vi "Read tag.vi"(8 "error in (no error)":errorcluster, 11 "current tag file io module runtime in":refnum<class "current tag file io module runtime.lvclass">) -> (0 "error out":errorcluster, 2 "tag":T1[](array[typedef]), 3 "current tag file io module runtime out":refnum<class "current tag file io module runtime.lvclass">)   [LabVIEW 2013, in "current tag file io module runtime.lvclass"]
uses:
  current tag file io module runtime.lvclass
  current tag file io configuration.ctl
  <vilib>/NI/Tag Bus/tag/Data Type.ctl
  current tag file io module runtime.lvclass/current tag file io module runtime.ctl
  <vilib>/NI/Tag Bus/tag/tag descriptor.lvclass
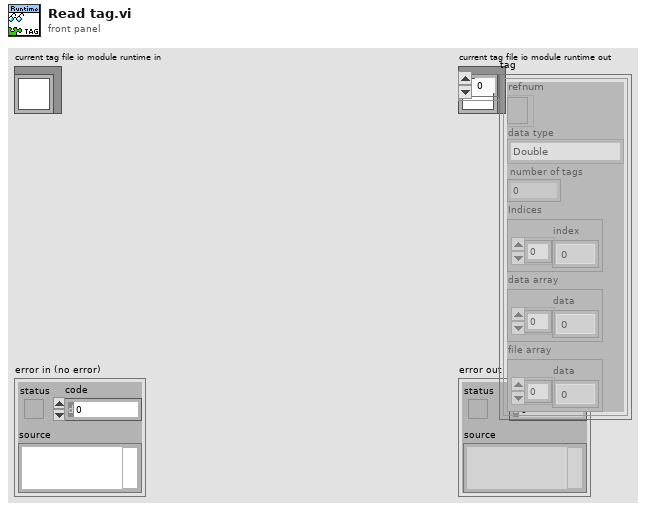
[diagram p1: front panel]
types:
  T1 = typedef "current tag file io module runtime.lvclass/current tag file io configuration.ctl" = cluster{"refnum":refnum<file>, "data type":T2, "number of tags":i32, "Indices":cluster{"index":i32[]}, "data array":cluster{"data":dbl[]}, "file array":cluster{"data":dbl[]}}
  T2 = typedef "tag bus.lvlib/tag descriptor.lvclass/Data Type.ctl" = enum16{"Double", "Single", "I64", "I32", "I16", "I8", "U64", "U32", "U16", "U8", "Boolean", "String", "Array of Double", "Array of Single", "Array of I64", "Array of I32", "Array of I16", "Array of I8", "Array of U64", "Array of U32", "Array of U16", "Array of U8", "Array of Boolean", "Array of String"}
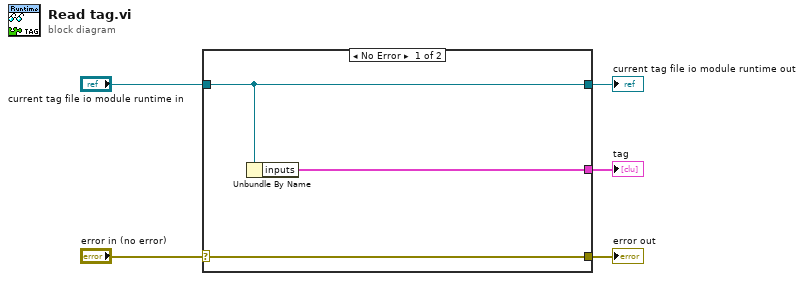
[diagram p0: block diagram]
diagram:
  n1 = case shown="No Error" "error in (no error)" {
    selector: "error in (no error)" -> [w8 w9]
    tunnel: [w8 w9] -> w4
    tunnel: [w7 w10] -> w2
    tunnel: "current tag file io module runtime in" -> [w7 w10]
    tunnel: [w6 _] -> w1
    frame No Error {
      n2 = Unbundle By Name(w7) -> ("inputs"=w6:T1[])
    }
    frame Error {
    }
  }
  "error out" <- w4
  "current tag file io module runtime out" <- w2
  "tag" <- w1
